vi "Wheel Controls.vi"   [LabVIEW 2012]
uses:
  <vilib>/Rock Robotics/WPI/Joystick/WPI_JoystickGetSetRefNum.vi
  <vilib>/Rock Robotics/WPI/Solenoid/Deprecated/WPI_SolenoidSetBool.vi
types:
  T1 = typedef "WPI_JoystickDevRef.ctl" = cluster{"Device":T2}
  T2 = typedef "WPI_JoystickDeviceEnum.ctl" = enum16{"USB 1", "USB 2", "USB 3", "USB 4", "Kinect 1", "Kinect 2"}
  T3 = typedef "WPI_SolenoidDevRef.ctl" = cluster{"DevStatus":errorcluster, "Solenoid Module":T4, "Forward Solenoid Channel":T5, "Reverse Solenoid Channel":T5}
  T4 = typedef "FPGA_TypedefSolenoidModule.ctl" = enum16{"Solenoid Module 1", "Solenoid Module 2"}
  T5 = typedef "WPI_SolenoidChannel.ctl" = enum8{"Solenoid 1", "Solenoid 2", "Solenoid 3", "Solenoid 4", "Solenoid 5", "Solenoid 6", "Solenoid 7", "Solenoid 8", "Invalid"}
  T6 = typedef "WPI_JoystickButtonState.ctl" = cluster{"Button 1":bool, "Button 2":bool, "Button 3":bool, "Button 4":bool, "Button 5":bool, "Button 6":bool, "Button 7":bool, "Button 8":bool, "Button 9":bool, "Button 10":bool, "Button 11":bool, "Button 12":bool}
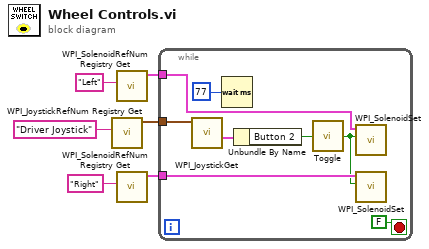
[diagram p0: block diagram]
diagram:
  n1 = call <vilib>:"WPI_JoystickRefNum Registry Get.vi"("refnum name"="Driver Joystick") -> ("JoystickDevRef"=w4:T1)  [unwired: 9 in, 1 out]
  n2 = call <vilib>:"WPI_SolenoidRefNum Registry Get.vi"("refnum name"="Left") -> ("SolenoidDevRef"=w1:T3)  [unwired: 9 in, 1 out]
  n3 = call <vilib>:"WPI_SolenoidRefNum Registry Get.vi"("refnum name"="Right") -> ("SolenoidDevRef"=w2:T3)  [unwired: 9 in, 1 out]
  n4 = while {
    tunnel: w4 -> [w12]
    tunnel: w2 -> [w11]
    tunnel: w1 -> [w10]
    stop <- FALSE stop-if-true
    n5 = call <vilib>:"WPI_JoystickGet.vi"("JoystickDevRef"=w12) -> ("Buttons"=w9:T6)  [unwired: 4 in, 2 out]
    n6 = Wait (ms)(milliseconds to wait=u32 77) -> ()  [unwired: 1 out]
    n7 = Unbundle By Name(w9) -> ("Button 2"=w8:bool)
    n8 = call "Toggle.vi"("Input"=w8) -> ("Output"=w7:bool)
    n9 = call-poly <vilib>:"WPI_SolenoidSet.vi"("Value"=w7, "SolenoidDevRef"=w10) -> ()  [unwired: 8 in, 2 out]
    n10 = call-poly <vilib>:"WPI_SolenoidSet.vi"("Value"=w7, "SolenoidDevRef"=w11) -> ()  [unwired: 8 in, 2 out]
  }
